vi "getImageDST.vi"(8 "error in (no error)":errorcluster, 11 "ax5 in":refnum<class "ax5.lvclass">) -> (0 "error out":errorcluster, 2 "Image":T1, 3 "ax5 out":refnum<class "ax5.lvclass">)   [LabVIEW 2017, in "ax5.lvclass"]
uses:
  ax5.lvclass
  <vilib>/vision/Image Controls.llb/IMAQ Image.ctl
  ax5.lvclass/ax5.ctl
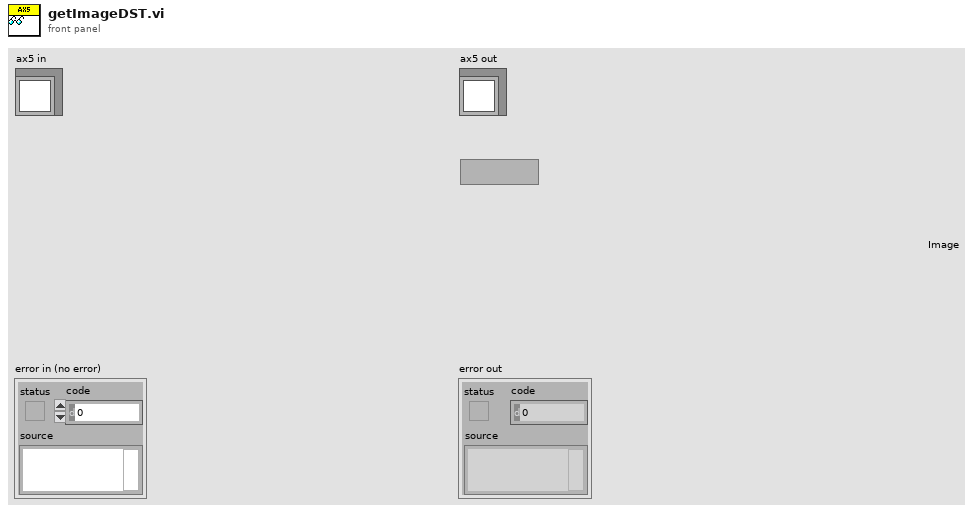
[diagram p1: front panel]
types:
  T1 = typedef "IMAQ Image.ctl" = refnum<image>
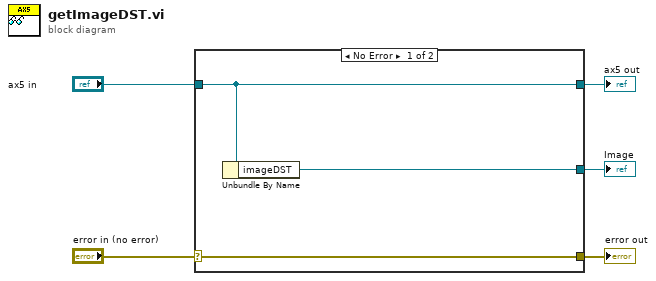
[diagram p0: block diagram]
diagram:
  n1 = case shown="No Error" "error in (no error)" {
    selector: "error in (no error)" -> [w8 w9]
    tunnel: [w8 w9] -> w4
    tunnel: [w7 w10] -> w2
    tunnel: "ax5 in" -> [w7 w10]
    tunnel: [w6 _] -> w1
    frame No Error {
      n2 = Unbundle By Name(w7) -> ("imageDST"=w6:T1)
    }
    frame Error {
    }
  }
  "error out" <- w4
  "ax5 out" <- w2
  "Image" <- w1
